vi "Test-Trace Controller.vi"() -> ()   [LabVIEW 2014]
uses:
  Robot Actor Framework/Trace/Trace Controller Class/Config.ctl
  Comp Robot/Comp Trace Controller/Comp Trace Controller Class/Comp Trace Controller.lvclass
  <vilib>/ActorFramework/Message Enqueuer/Message Enqueuer.lvclass/Message Enqueuer.ctl
  <vilib>/ActorFramework/Message Enqueuer/Enqueue.vi
  <vilib>/ActorFramework/Message Priority Queue/Priority Enqueue.vi
  <vilib>/ActorFramework/Stop Msg/Stop Msg.lvclass
  <vilib>/ActorFramework/Actor/Actor.lvclass
  Robot Actor Framework/Trace/Trace Controller Class/Trace Controller.lvclass
panel:
  in  "stop":bool
  in  "Config":T1={"Folder Pattern"="/media/sd%s1", "Starting Letter Position"=1, "Min Free Space (MB)"=50.0, "Max Folders to Check"=10, "Trace Level"=enum."Debug"} {"Min Free Space (MB)" format="%#_13g"}
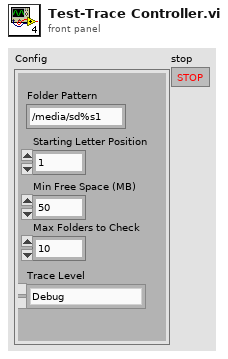
[diagram p1: front panel]
types:
  T1 = typedef "Robot Actor Framework.lvlib/Trace.lvlib/Trace Controller.lvclass/Config.ctl" = cluster{"Folder Pattern":string, "Starting Letter Position":i32, "Min Free Space (MB)":dbl, "Max Folders to Check":u32, "Trace Level":enum16{"Critical", "Error", "Warning", "Informational", "Debug"}}
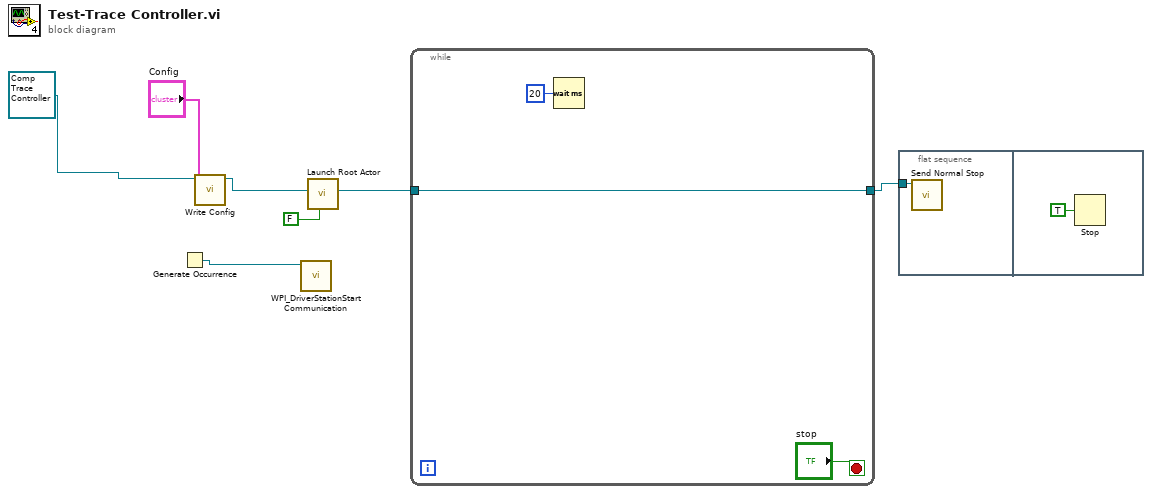
[diagram p0: block diagram]
diagram:
  n1 = Generate Occurrence() -> (w1:refnum<k4>)
  n2 = call-dynamic "Write Config.vi"("Config"="Config", "Trace Controller in"=refnum<class "Comp Trace Controller.lvclass"> refnum ("Comp Trace Controller.lvlib:Comp Trace Controller.lvclass")) -> ("Trace Controller out"=w5:refnum<class "Comp Trace Controller.lvclass">)  [unwired: 8 in, 1 out]
  n3 = call <vilib>:"WPI_DriverStationStart Communication.vi"("occurrence"=w1) -> ()  [unwired: 1 in, 10 out]
  n4 = call <vilib>:"Launch Root Actor.vi"("Open Actor Core front panel? (F)"=FALSE, "Actor"=w5) -> ("Actor's Enqueuer"=w3:refnum<class "Message Enqueuer.lvclass">)  [unwired: 8 in, 1 out]
  n5 = while {
    tunnel: w3 -> [w8]
    tunnel: [w8] -> w2
    stop <- "stop" stop-if-true
    n6 = Wait (ms)(milliseconds to wait=u32 20) -> ()  [unwired: 1 out]
  }
  n7 = flat-sequence {
    tunnel: w2 -> [w11]
    frame #0 {
      n8 = call <vilib>:"Send Normal Stop.vi"("Message Enqueuer"=w11) -> ()  [unwired: 10 in, 1 out]
    }
    frame #1 {
      n9 = Stop(stop? (T)=TRUE) -> ()
    }
  }
